vi "nCarnot.vi"(10 "Temp hot":dbl, 11 "Numeric":dbl) -> (3 "nCarrot":dbl)   [LabVIEW 2020]
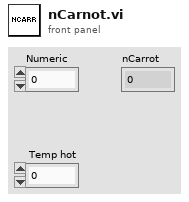
[diagram p1: front panel]
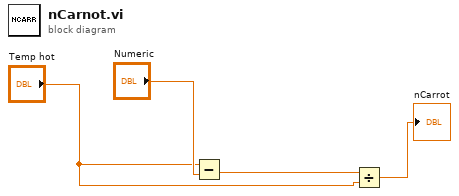
[diagram p0: block diagram]
diagram:
  n1 = Subtract(x="Temp hot", y="Numeric") -> (x-y=w2:dbl)
  n2 = Divide(x=w2, y="Temp hot") -> (x/y=→"nCarrot":dbl)
